vi "setXML.vi"(8 "error in":errorcluster, 9 "Controls filtered":cluster{"name":string, "type desc":i16[]}[](array[cluster]), 10 "Indicators filtered":cluster{"name":string, "type desc":i16[]}[](array[cluster]), 11 "connection ID in":refnum<k5>) -> (0 "error out":errorcluster, 3 "connection ID out":refnum<k5>)   [LabVIEW 2010]
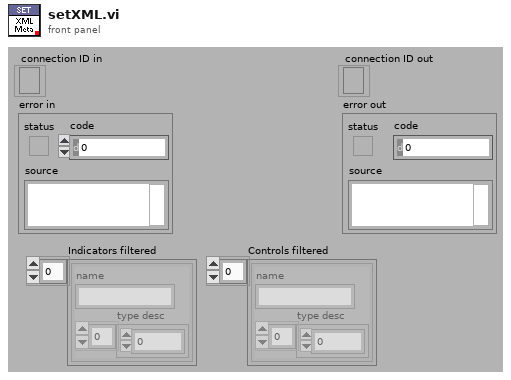
[diagram p1: front panel]
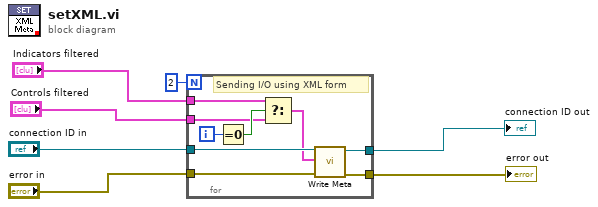
[diagram p0: block diagram]
diagram:
  n1 = for {
    N: 2 -> [_]
    tunnel: "error in" -> [w16]
    tunnel: "connection ID in" -> [w15]
    tunnel: [w14] -> w4
    tunnel: [w13] -> w3
    tunnel: "Indicators filtered" -> [w10]
    tunnel: "Controls filtered" -> [w9]
    i -> [w12]
    # "Sending I/O using XML form"
    n2 = Equal To 0?(x=w12) -> (x = 0?=w11:bool)
    n3 = Select(t=w10, s=w11, f=w9) -> (s? t:f=w8:cluster{"name":string, "type desc":i16[]}[])
    n4 = call "Write Meta.vi"("error in"=w16, "Variables"=w8, "connection ID"=w15) -> ("error out"=w13:errorcluster, "connection ID out"=w14:refnum<k5>)  [unwired: 7 out]
  }
  "connection ID out" <- w4
  "error out" <- w3
